vi "Exemple_Random_Projection_Johnson.vi"() -> ()   [LabVIEW 2020]
panel:
  in  "johnson_lindenstrauss_min_dim":cluster{"n_samples":i32[], "eps":dbl[]}={"n_samples"=[1000000], "eps"=[0.5, 0.1, 0.01]} {"eps" min=0.0 max=1.0}
  out "Data":T1
  out "error out":errorcluster caption="sortie d'erreur"
  in  "error in":errorcluster caption="entrée d'erreur"
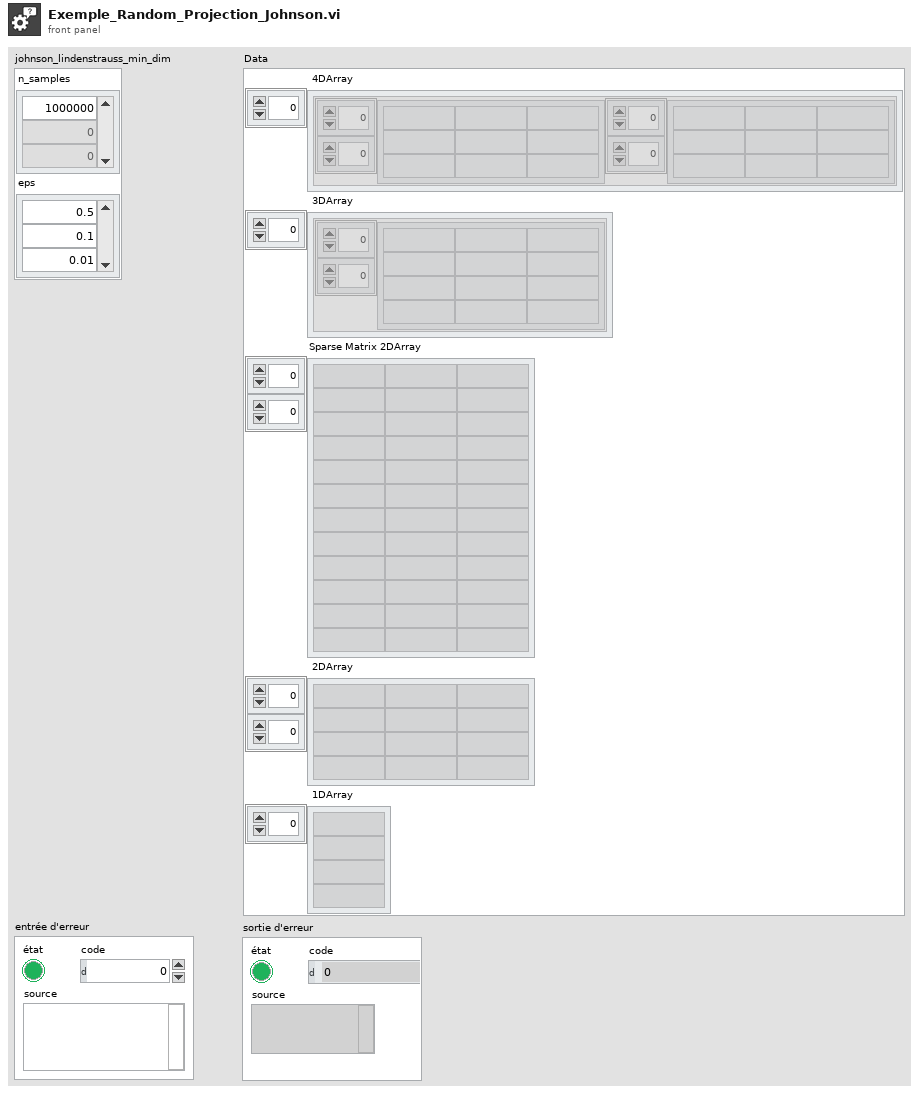
[diagram p1: front panel]
types:
  T1 = cluster{" 4DArray":cluster{"1":string[][], "2":string[][]}[], " 3DArray":cluster{"Tableau":string[][]}[], "Sparse Matrix 2DArray":string[][], " 2DArray":string[][], " 1DArray":string[]}
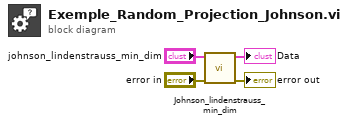
[diagram p0: block diagram]
diagram:
  n1 = call "Johnson_lindenstrauss_min_dim.vi"("error in"="error in", "johnson_lindenstrauss_min_dim"="johnson_lindenstrauss_min_dim") -> ("error out"=→"error out":errorcluster, "Data"=→"Data":T1)  [unwired: 8 in]
